vi "Get Latest Scan Build.vi"() -> ()   [LabVIEW 2013]
uses:
  <vilib>/FTP/NI_FTP.lvlib
panel:
  out "error out":errorcluster
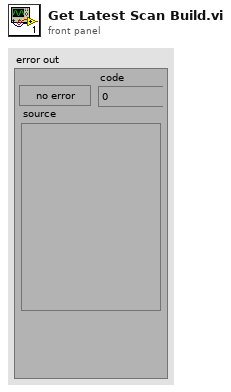
[diagram p1: front panel]
types:
  T1 = cluster{"remote path":string, "local path":path, "binary":bool}
  T2 = typedef "NI_FTP.lvlib/FTP Session.ctl" = refnum<k5>
  T3 = typedef "NI_FTP.lvlib/FTP File Info.ctl" = cluster{"type":enum16{"unknown", "file", "dir", "link"}, "permissions":string, "owner":string, "group":string, "size":i32, "date":string, "name":string, "link name":string}
  T4 = cluster{"remote path":string, "local path":path, "binary":bool}[]
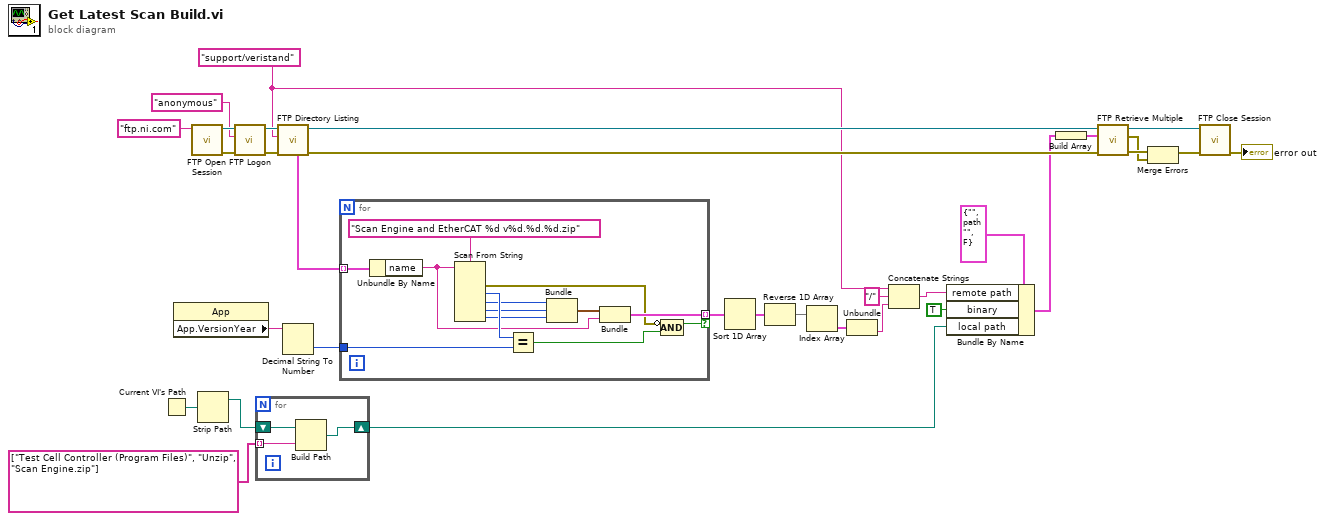
[diagram p0: block diagram]
diagram:
  w15 = "support/veristand" ("directory path")
  n1 = Current VI's Path() -> (path=w5:path)
  n2 = property class="App"() -> ("App.VersionYear"=w24:string)  [unwired: 2 in, 2 out]
  n3 = call <vilib>:"FTP Open Session.vi"("address"="ftp.ni.com") -> ("error out"=w31:errorcluster, "ftp session"=w28:T2)  [unwired: 7 in, 2 out]
  n4 = Strip Path(path=w5) -> (stripped path=w4:path)  [unwired: 1 out]
  n5 = call <vilib>:"FTP Logon.vi"("error in (no error)"=w31, "user"="anonymous", "ftp session"=w28) -> ("error out"=w29:errorcluster, "ftp session out"=w27:T2)  [unwired: 5 in, 2 out]
  n6 = for {
    shift-right: [w34] -> w2
    shift-left: w4 -> [w35]
    tunnel: string[] ["Test Cell Controller (Program Files)", "Unzip", "Scan Engine.zip"] -> [w33] mode=indexing
    n7 = Build Path(base path=w35, name or relative path=w33) -> (appended path=w34:path)
  }
  n8 = call <vilib>:"FTP Directory Listing.vi"("error in (no error)"=w29, "directory path"=w15, "ftp session"=w27) -> ("error out"=w18:errorcluster, "ftp session out"=w20:T2, "dir list"=w25:T3[])  [unwired: 4 in, 2 out]
  n9 = Decimal String To Number(string=w24) -> (number=w23:i32)  [unwired: 2 in, 1 out]
  n10 = for {
    tunnel: w25 -> [w48] mode=indexing
    tunnel: w23 -> [w45]
    tunnel: [w39] -> w22 mode=indexing if=w38
    n11 = Unbundle By Name(w48) -> ("name"=w40:string)
    n12 = Scan From String(format string="Scan Engine and EtherCAT %d v%d.%d.%d.zip", input string=w40) -> (error out=w36:errorcluster, output 1=w46:i32, output 2=w44:i32, output 3=w43:i32, output 4=w42:i32)  [unwired: 6 in, 2 out]
    n13 = Equal?(x=w46, y=w45) -> (x = y?=w37:bool)
    n14 = Bundle(w44, w43, w42) -> (w41:cluster{i32, i32, i32})  [unwired: 1 in]
    n15 = Bundle(w41, "name"=w40) -> (w39:cluster{cluster{i32, i32, i32}, "name":string})  [unwired: 1 in]
    n16 = Compound Arithmetic op=AND(invert w36, w37) -> (w38:bool)
  }
  n17 = Sort 1D Array(array=w22) -> (sorted array=w21:cluster{cluster{i32, i32, i32}, "name":string}[])
  n18 = Reverse 1D Array(array=w21) -> (reversed array=w17:cluster{cluster{i32, i32, i32}, "name":string}[])
  n19 = Index Array(array=w17) -> (element=w14:cluster{cluster{i32, i32, i32}, "name":string})  [unwired: 1 in]
  n20 = Unbundle(w14) -> ("name"=w13:string)  [unwired: 1 out]
  n21 = Concatenate Strings(w15, "/" ("string"), w13) -> (w6:string)
  n22 = Bundle By Name(cluster=T1 {"remote path"="", "local path"=path "", "binary"=FALSE} ("transfer spec"), "remote path"=w6, "binary"=TRUE, "local path"=w2) -> (w12:T1)
  n23 = Build Array(w12) -> (w11:T4)
  n24 = call <vilib>:"FTP Retrieve Multiple.vi"("error in (no error)"=w18, "file specifications"=w11, "ftp session"=w20) -> ("error out"=w9:errorcluster, "file errors"=w8:errorcluster[], "ftp session out"=w19:T2)  [unwired: 5 in, 1 out]
  n25 = Merge Errors(w9, w8) -> (w10:errorcluster)
  n26 = call <vilib>:"FTP Close Session.vi"("error in (no error)"=w10, "ftp session"=w19) -> ("error out"=→"error out":errorcluster)  [unwired: 6 in, 3 out]
